vi "Actor Core.vi"(8 "error in":errorcluster, 11 "AnalogInput in":refnum<class "AnalogInput.lvclass">) -> (0 "error out":errorcluster, 3 "Actor out":refnum<class "Actor.lvclass">)   [LabVIEW 2019, in "AnalogInput.lvlib" / "AnalogInput.lvclass"]
uses:
  Library/AnalogInput.lvclass
  C:/Users/Public/Documents/Development/builds/Instruments/Instruments.lvlibp/Library/Instruments.lvclass
  builds/Engine/Actor Framework.lvlibp/1abvi3w/vi.lib/ActorFramework/Actor/Actor.lvclass
  Custom Controls/User Trigger Settings.ctl
  Custom Controls/Trigger_Slope.ctl
  Library/AnalogInput.lvclass/AnalogInput.ctl
  AnalogInput Messages/Write User Trigger Settings Msg/Write User Trigger Settings Msg.lvclass/Write User Trigger Settings Msg.ctl
  AnalogInput Messages/Write Trigger Source Msg/Write Trigger Source Msg.lvclass/Write Trigger Source Msg.ctl
  Accessors/Read Num Channels.vi
  Accessors/Write Timeout Reference.vi
  Accessors/Write User Trigger Settings Reference.vi
  Accessors/Write Measured Table Reference.vi
  Accessors/GUI/Write Trig Src Ref.vi
  builds/Instruments/Instruments.lvlibp/Accessors/Write Graph_Ref.vi
  builds/Instruments/Instruments.lvlibp/Accessors/Write Snapshot Refnum.vi
  Append Digital Trigger Name.vi
  builds/Engine/Actor Framework.lvlibp/1abvi3w/vi.lib/ActorFramework/Message Enqueuer/Enqueue.vi
  builds/Engine/Actor Framework.lvlibp/1abvi3w/vi.lib/ActorFramework/Message Enqueuer/Message Enqueuer.lvclass
  AnalogInput Messages/Write User Trigger Settings Msg/Write User Trigger Settings Msg.lvclass
  AnalogInput Messages/Write Trigger Source Msg/Write Trigger Source Msg.lvclass
  builds/Instruments/Instruments.lvlibp/Library/Instruments.lvclass
  builds/Instruments/Instruments.lvlibp/Instruments Messages/Take Snapshot Msg/Take Snapshot Msg.lvclass
panel:
  out "Timed Out":bool
  in  "Active Device":u16(ring)
  in  "Hi Spd Snap":bool
  in  "Hide Plots":bool=TRUE
  in  "User Trigger Settings":T1={"Timeout"=0.0, "Level"=0.0, "Slope"=enum."Falling", "samples per channel"=1000, "Sample Rate (10k)"=10000.0, "pretrigger samples"=50}
  in  "Trigger Source":u16(ring)
  in  "View":enum16{"Continuous", "Snapshot", "Table"}(ring)
  out "Display Format":enum32{"Continuous", "Snapshot", "Table"}(tab)
  out "Continuous Plot":waveform(dbl)[](graph)
  out "Delta(ms)":dbl
  out "Snapshot Plot":waveform(dbl)[](graph)
  out "Measured Table":i32(listbox)
  # "Trigger Settings"
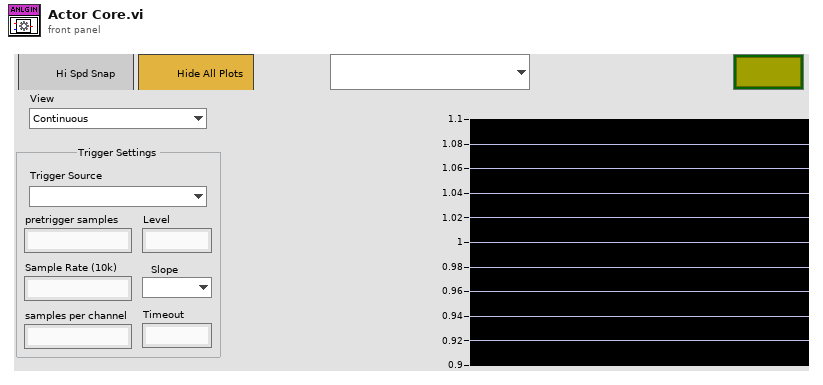
[diagram p1: front panel]
types:
  T1 = typedef "AnalogInput.lvlib/AnalogInput.lvclass/User Trigger Settings.ctl" = cluster{"Timeout":dbl, "Level":dbl, "Slope":T2, "samples per channel":i32, "Sample Rate (10k)":dbl, "pretrigger samples":u32}
  T2 = typedef "AnalogInput.lvlib/AnalogInput.lvclass/Trigger_Slope.ctl" = enum16{"Rising", "Falling"}
  T3 = cluster{"Pnl Actor":refnum<event-registration>, "Event Registration Refnum":refnum<event-registration>}
  T4 = typedef "LVCursorListTypeDef.ctl" = cluster{"Name":string, "Color":u32, "Style":u8, "Point Style":u8, "Name Visible":bool, "Allow Drag":bool, "Cursor Mode":u32, "Plot":i32, "Index":i32, "Position":cluster{"X":dbl, "Y":dbl}, "X Scale":u32, "Y Scale":u32, "Watch Plots":i32[], "Watch All Plots":bool, "Plot Area":i32, "Label Offset":cluster{"X":dbl, "Y":dbl}}[]
  T5 = cluster{"Name":string, "Color":u32, "Style":u8, "Point Style":u8, "Name Visible":bool, "Allow Drag":bool, "Cursor Mode":u32, "Plot":i32, "Index":i32, "Position":cluster{"X":dbl, "Y":dbl}, "X Scale":u32, "Y Scale":u32, "Watch Plots":i32[], "Watch All Plots":bool, "Plot Area":i32, "Label Offset":cluster{"X":dbl, "Y":dbl}}
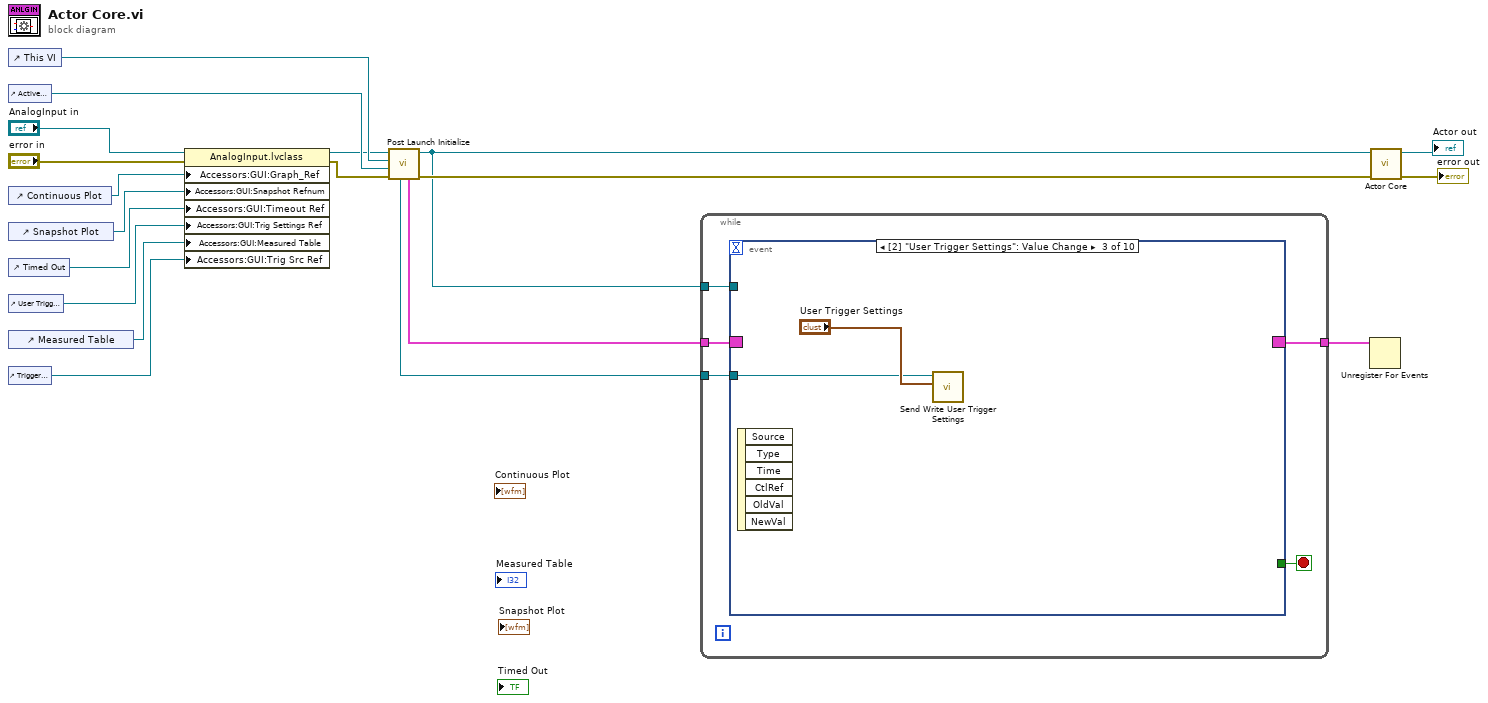
[diagram p0: block diagram]
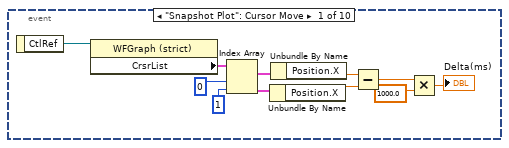
[diagram p2: hidden frame]
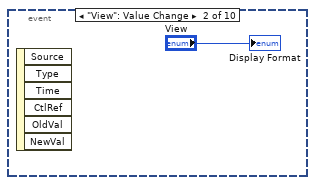
[diagram p3: hidden frame]
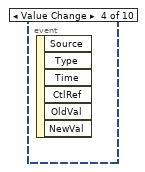
[diagram p4: hidden frame]
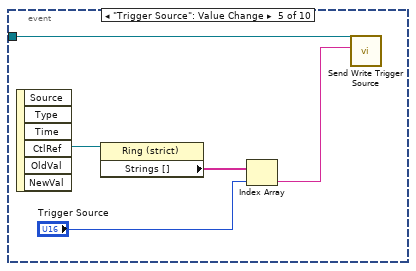
[diagram p5: hidden frame]
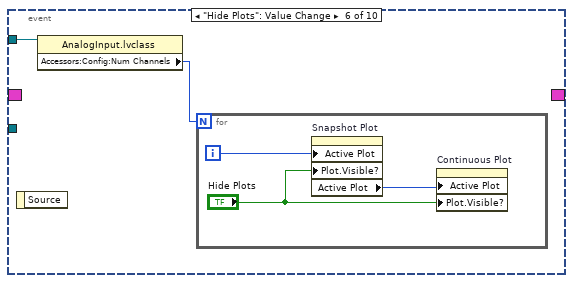
[diagram p6: hidden frame]
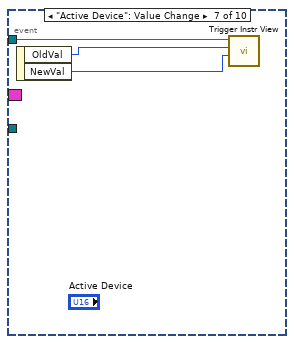
[diagram p7: hidden frame]
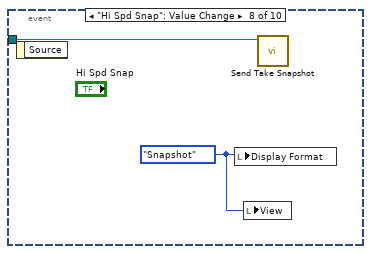
[diagram p8: hidden frame]
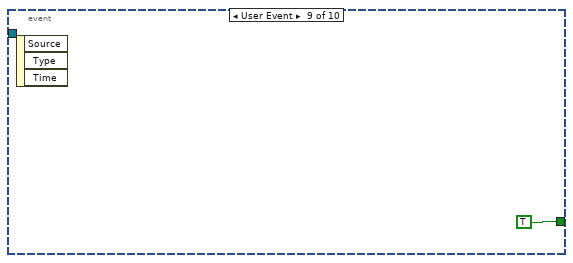
[diagram p9: hidden frame]
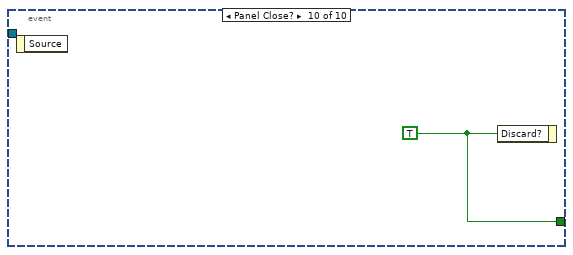
[diagram p10: hidden frame]
diagram:
  n1 = control-ref of="This VI"() -> (w19:refnum<vi>)
  n2 = control-ref of="Active Device"() -> (w18:refnum<vi>)
  n3 = control-ref of="Continuous Plot"() -> (w8:refnum<vi>)
  n4 = control-ref of="Snapshot Plot"() -> (w7:refnum<vi>)
  n5 = control-ref of="Timed Out"() -> (w6:refnum<vi>)
  n6 = control-ref of="User Trigger Settings"() -> (w5:refnum<vi>)
  n7 = control-ref of="Measured Table"() -> (w4:refnum<vi>)
  n8 = control-ref of="Trigger Source"() -> (w3:refnum<vi>)
  n9 = property class="AnalogInput.lvclass"(reference="AnalogInput in", error in="error in", "Accessors:GUI:Graph_Ref"=w8, "Accessors:GUI:Snapshot Refnum"=w7, "Accessors:GUI:Timeout Ref"=w6, "Accessors:GUI:Trig Settings Ref"=w5, "Accessors:GUI:Measured Table"=w4, "Accessors:GUI:Trig Src Ref"=w3) -> (reference out=w16:refnum<class "AnalogInput.lvclass">, error out=w1:errorcluster)
  n10 = call "Post Launch Initialize.vi"("error in"=w1, "Active Device"=w18, "GUI Reference"=w19, "Instruments in"=w16) -> ("error out"=w13:errorcluster, "Instruments out"=w9:refnum<class "AnalogInput.lvclass">, "Registered Events"=w12:T3, "Self Enqueuer"=w10:refnum<class "Message Enqueuer.lvclass">)  [unwired: 4 in]
  n11 = while {
    tunnel: w12 -> [w23]
    tunnel: [w22] -> w11
    tunnel: w10 -> [w20]
    tunnel: w9 -> [w21]
    stop <- w24 stop-if-true
    n12 = event shown="[2] \"User Trigger Settings\": Value Change" {
      selector: w23 -> [_ _ _ _ _ _ _ _ _ _]
      dyn-events: [_ _ _ _ _ _ _ _ _ _] -> w22
      timeout: _ -> [_ _ _ _ _ _ _ _ _ _]
      tunnel: [_ _ _ _ _ _ _ _ TRUE ("stop") w56] -> w24
      tunnel: w20 -> [_ _ w37 _ w43 _ w52 w53 _ _]
      tunnel: [_ _ _ _ _ _ w52 _ _ _] -> _
      tunnel: w21 -> [_ _ _ _ _ w45 w51 _ _ _]
      event "Snapshot Plot": Cursor Move {
        n13 = event-data() -> ("CtlRef"=w25:refnum<vi>)  [unwired: 1 in]
        n14 = property on="Property Node" class="WFGraph (strict)"(reference=w25) -> ("CrsrList"=w35:T4)  [unwired: 1 in, 2 out]
        n15 = Index Array(array=w35, index #1=0 ("index"), index #2=1 ("index")) -> (element #1=w32:T5, element #2=w31:T5)
        n16 = Unbundle By Name(w31) -> ("Position.X"=w30:dbl)
        n17 = Unbundle By Name(w32) -> ("Position.X"=w29:dbl)
        n18 = Subtract(x=w29, y=w30) -> (x-y=w28:dbl)
        n19 = Multiply(x=w28, y=1000.0) -> (x*y=→"Delta(ms)":dbl)
      }
      event "View": Value Change {
        n20 = event-data() -> ()  [unwired: 1 in, 6 out]
        "Display Format" <- "View"
      }
      event Value Change {
        n21 = event-data() -> ()  [unwired: 1 in, 6 out]
        n22 = call "Send Write User Trigger Settings.vi"("User Trigger Settings"="User Trigger Settings", "Message Enqueuer"=w37) -> ()  [unwired: 8 in, 2 out]
      }
      event Value Change {
        n23 = event-data() -> ()  [unwired: 1 in, 6 out]
      }
      event "Trigger Source": Value Change {
        n24 = event-data() -> ("CtlRef"=w42:refnum<vi>)  [unwired: 1 in, 5 out]
        n25 = property class="Ring (strict)"(reference=w42) -> ("Strings []"=w41:string[])  [unwired: 1 in, 2 out]
        n26 = Index Array(array=w41, index="Trigger Source") -> (element=w39:string)
        n27 = call "Send Write Trigger Source.vi"("Trigger Source"=w39, "Message Enqueuer"=w43) -> ()  [unwired: 8 in, 2 out]
      }
      event "Hide Plots": Value Change {
        n28 = event-data() -> ()  [unwired: 1 in, 1 out]
        n29 = property class="AnalogInput.lvclass"(reference=w45) -> ("Accessors:Config:Num Channels"=w44:u32)  [unwired: 1 in, 2 out]
        n30 = for {
          N: w44 -> [_]
          i -> [w47]
          n31 = property on="Snapshot Plot" class="WFGraph (strict)"("Active Plot"=w47, "Plot.Visible?"="Hide Plots") -> ("Active Plot"=w46:u32)  [unwired: 2 in, 2 out]
          n32 = property on="Continuous Plot" class="WFChart (strict)"("Active Plot"=w46, "Plot.Visible?"="Hide Plots") -> ()  [unwired: 2 in, 2 out]
        }
      }
      event "Active Device": Value Change {
        n33 = event-data() -> ("OldVal"=w50:u16, "NewVal"=w49:u16)  [unwired: 1 in]
        n34 = call "Trigger Instr View.vi"("New Value"=w49, "Old Value"=w50, "Instruments in"=w51) -> ()  [unwired: 7 in, 2 out]
      }
      event "Hi Spd Snap": Value Change {
        w54 = enum16{"Continuous", "Snapshot", "Table"}."Snapshot" ("View")
        n35 = event-data() -> ()  [unwired: 1 in, 1 out]
        n36 = local write "Display Format"(w54) -> ()
        n37 = local write "View"(w54) -> ()
        n38 = call "Send Take Snapshot.vi"("Message Enqueuer"=w53) -> ()  [unwired: 9 in, 2 out]
      }
      event User Event {
        n39 = event-data() -> ()  [unwired: 1 in, 3 out]
      }
      event Panel Close? {
        w56 = TRUE ("Discard?")
        n40 = event-data() -> ()  [unwired: 1 in, 1 out]
        n41 = event-data("Discard?"=w56) -> ()  [unwired: 1 in, 1 out]
      }
    }
  }
  n42 = Unregister For Events(event registration refnum=w11) -> ()  [unwired: 1 in, 1 out]
  n43 = call-parent "Actor Core.vi"("error in"=w13, "Instruments in"=w9) -> ("error out"=→"error out":errorcluster, "Actor out"=→"Actor out":refnum<class "Actor.lvclass">)  [unwired: 8 in]
